vi "Convert Digital to Channel Settings.vi"(10 "channel default values":dbl[](array[numeric]), 11 "channel names":string[](array[string])) -> (3 "channel settings":T1[](array[typedef]))   [LabVIEW 2020, in "Scan Engine Scripting.lvlib"]
uses:
  Scan Engine Scripting.lvlib
  Modules/Mode Classes/Controls/digital channel settings.ctl
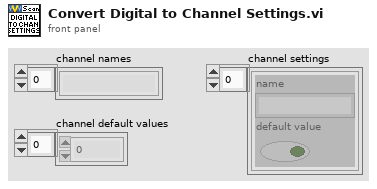
[diagram p1: front panel]
types:
  T1 = typedef "Scan Engine Scripting.lvlib/digital channel settings.ctl" = cluster{"name":string, "default value":bool}
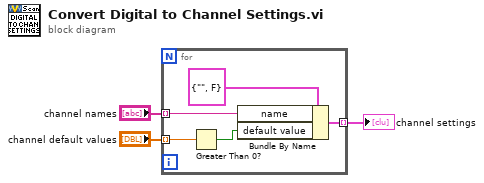
[diagram p0: block diagram]
diagram:
  n1 = for {
    tunnel: "channel names" -> [w7] mode=indexing
    tunnel: "channel default values" -> [w6] mode=indexing
    tunnel: [w4] -> w3 mode=indexing
    n2 = Greater Than 0?(x=w6) -> (x > 0?=w5:bool)
    n3 = Bundle By Name(cluster=T1 {"name"="", "default value"=FALSE} ("channel settings"), "name"=w7, "default value"=w5) -> (w4:T1)
  }
  "channel settings" <- w3
